vi "Destroy.vi"(8 "error in (no error)":errorcluster, 11 "Mock Result Observer in":refnum<class "Mock Result Observer.lvclass">) -> (0 "error out":errorcluster)   [LabVIEW 2020, in "Mock Result Observer.lvclass"]
uses:
  Mock Result Observer.lvclass
  Mock Result Observer.lvclass/Mock Result Observer.ctl
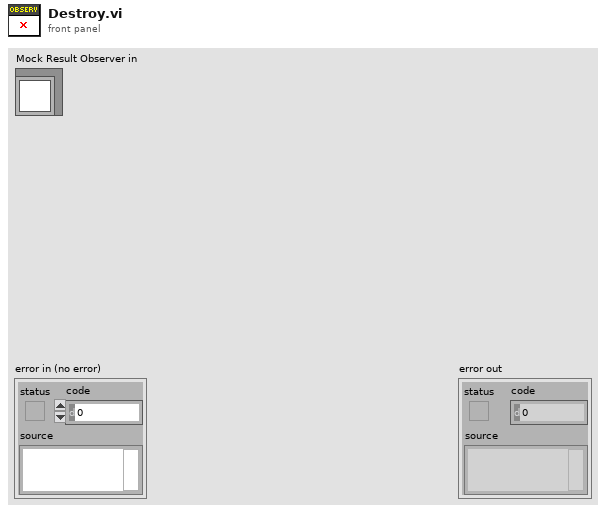
[diagram p1: front panel]
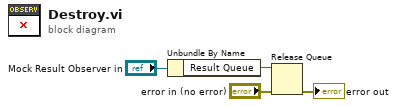
[diagram p0: block diagram]
diagram:
  n1 = Unbundle By Name("Mock Result Observer in") -> ("Result Queue"=w1:refnum<queue>)
  n2 = Release Queue(queue=w1, error in (no error)="error in (no error)") -> (error out=→"error out":errorcluster)  [unwired: 1 in, 2 out]
